vi "log analysis_gps.vi"() -> ()   [LabVIEW 2019] (continued)
-1.551528\t-0.373254\t-10.328419\t0.302000\t0.041000\n\t\n15:17:08.7\tlog_raw\tgps_raw\t#DUALANTENNAHEADINGA,USB3,0,50.0,FINESTEERING,2107,281846.700,02000000,d426,15824;SOL_COMPUTED,L1_FLOAT,-1.000000000,97.773071289,12.519289017,0.0,360.000000000,180.000000000,\"631T\",20,6,6,3,04,00,20,01*fc76e214\n\tsystem status\tnormal 2 27.800000 0 0\trobot status\t187.429657\t118.350310\t7.996000\t-1.404471\t-0.508241\t-9.481773\t0.290000\t0.043000\n\t\n15:17:09.2\tlog_raw\tgps_raw\t#DUALANTENNAHEADINGA,USB3,0,48.5,FINESTEERING,2107,281847.200,02000000,d426,15824;SOL_COMPUTED,L1_FLOAT,-1.000000000,99.566589355,2.463819742,0.0,360.000000000,180.000000000,\"631T\",20,6,6,3,04,00,20,01*aa8a8936\n\tsystem status\tnormal 2 27.900000 0 0\trobot status\t187.566793\t118.321024\t7.994500\t-1.416606\t-0.450416\t-8.715947\t0.329000\t-0.016000\n\t\n15:17:09.7\tlog_raw\tgps_raw\t#DUALANTENNAHEADINGA,USB3,0,48.5,FINESTEERING,2107,281847.700,02000000,d426,15824;SOL_COMPUTED,L1_FLOAT,-1.000000000,101.704925537,-0.791503906,0.0,360.000000000,180.000000000,\"631T\",21,6,6,3,04,00,20,01*ba1d7434\n\tsystem status\tnormal 2 28.000000 0 0\trobot status\t187.708819\t118.292371\t7.992200\t-1.444500\t-0.439049\t-8.038629\t0.312000\t-0.001000\n\t\n15:17:10.2\tlog_raw\tgps_raw\t#DUALANTENNAHEADINGA,USB3,0,48.0,FINESTEERING,2107,281848.200,02000000,d426,15824;SOL_COMPUTED,NARROW_FLOAT,-1.000000000,68.873619080,-13.291412354,0.0,268.060089111,180.000000000,\"631T\",21,7,7,5,04,00,20,03*0971a231\n\tsystem status\tnormal 2 28.000000 0 0\trobot status\t187.851802\t118.263763\t7.990800\t-1.419717\t-0.363643\t-7.607378\t0.249000\t0.089000\n\t\n15:17:10.7\tlog_raw\tgps_raw\t#DUALANTENNAHEADINGA,USB3,0,48.0,FINESTEERING,2107,281848.700,02000000,d426,15824;SOL_COMPUTED,NARROW_FLOAT,-1.000000000,68.326225281,-12.809478760,0.0,266.431640625,180.000000000,\"631T\",22,7,7,5,04,00,20,03*e2c6400d\n\tsystem status\tnormal 2 28.000000 0 0\trobot status\t187.993908\t118.234860\t7.989100\t-1.318472\t-0.217870\t-7.309537\t0.279000\t0.046000\n\t\n15:17:11.2\tlog_raw\tgps_raw\t#DUALANTENNAHEADINGA,USB3,0,49.0,FINESTEERING,2107,281849.200,02000000,d426,15824;SOL_COMPUTED,L1_FLOAT,-1.000000000,90.585990906,2.083147287,0.0,360.000000000,180.000000000,\"631T\",19,6,6,3,04,00,20,01*dc534f3f\n\tsystem status\tnormal 2 28.100000 0 0\trobot status\t188.136584\t118.206878\t7.987700\t-1.302740\t-0.167404\t-7.137371\t0.263000\t0.048000\n\t\n15:17:11.7\tlog_raw\tgps_raw\t\tsystem status\tnormal 2 28.100000 0 0\trobot status\t188.281681\t118.179408\t7.986200\t-1.424741\t-0.244800\t-7.144993\t0.355000\t-0.100000\n\t\n15:17:12.2\tlog_raw\tgps_raw\t\tsystem status\tnormal 2 28.100000 0 0\trobot status\t188.424376\t118.151727\t7.985000\t-1.444074\t-0.321672\t-7.277293\t0.280000\t0.006000\n\t\n15:17:12.7\tlog_raw\tgps_raw\t\tsystem status\tnormal 2 28.100000 0 0\trobot status\t188.565924\t118.124361\t7.984600\t-1.373448\t-0.224208\t-7.361017\t0.301000\t-0.011000\n\t\n15:17:13.2\tlog_raw\tgps_raw\t\tsystem status\tnormal 2 28.200000 0 0\trobot status\t188.708555\t118.095223\t7.983900\t-1.237162\t-0.173979\t-7.470326\t0.299000\t-0.027000\n\t\n15:17:13.7\tlog_raw\tgps_raw\t\tsystem status\tnormal 2 28.100000 0 0\trobot status\t188.846950\t118.066216\t7.984500\t-1.256970\t-0.201801\t-7.611888\t0.295000\t-0.025000\n\t\n15:17:14.2\tlog_raw\tgps_raw\t\tsystem status\tnormal 2 28.200000 0 0\trobot status\t188.990067\t118.035749\t7.985300\t-1.203931\t-0.250231\t-7.787271\t0.299000\t-0.026000\n\t\n15:17:14.7\tlog_raw\tgps_raw\t#DUALANTENNAHEADINGA,USB3,0,50.5,FINESTEERING,2107,281852.700,02000000,d426,15824;SOL_COMPUTED,L1_FLOAT,-1.000000000,102.741966248,-6.929687500,0.0,360.000000000,180.000000000,\"631T\",20,6,6,3,04,00,20,01*85f8aaaa\n\tsystem status\tnormal 2 28.100000 0 0\trobot status\t189.132338\t118.004982\t7.987500\t-1.054884\t-0.345405\t-7.976871\t0.298000\t-0.028000\n\t\n15:17:15.2\tlog_raw\tgps_raw\t#DUALANTENNAHEADINGA,USB3,0,48.0,FINESTEERING,2107,281853.200,02000000,d426,15824;SOL_COMPUTED,NARROW_FLOAT,-1.000000000,142.458068848,56.396076202,0.0,360.000000000,180.000000000,\"631T\",20,7,7,7,04,00,20,23*a5970788\n\tsystem status\tnormal 2 28.100000 0 0\trobot status\t189.287326\t117.973168\t7.989400\t-1.112733\t-0.467352\t-8.155902\t0.296000\t-0.018000\n\t\n15:17:15.7\tlog_raw\tgps_raw\t#DUALANTENNAHEADINGA,USB3,0,48.0,FINESTEERING,2107,281853.700,02000000,d426,15824;SOL_COMPUTED,NARROW_FLOAT,-1.000000000,133.951141357,46.090900421,0.0,360.000000000,180.000000000,\"631T\",20,7,7,7,04,00,20,23*158a3a24\n\tsystem status\tnormal 2 28.100000 0 0\trobot status\t189.431373\t117.943241\t7.991600\t-1.182526\t-0.406297\t-8.448718\t0.296000\t-0.020000\n\t\n15:17:16.2\tlog_raw\tgps_raw\t#INSPVAXA,USB3,0,49.5,FINESTEERING,2107,281854.250,02000000,471d,15824;INS_ALIGNMENT_COMPLETE,INS_RTKFIXED,37.37119259093,126.72297552525,7.9951,22.3000,-0.0458,0.2655,0.0156,-1.071259362,-0.181379499,98.712494459,0.4123,0.2982,0.5510,0.1098,0.0931,0.0772,0.1581,0.1591,4.8949,0f000001,0*3786ee92\n\tsystem status\tnormal 2 28.100000 0 0\trobot status\t189.594911\t117.907272\t7.995100\t-1.071259\t-0.181379\t-8.712494\t0.243000\t-0.107000\n\t\n15:17:16.7\tlog_raw\tgps_raw\t#INSPVAXA,USB3,0,49.5,FINESTEERING,2107,281854.750,02000000,471d,15824;INS_ALIGNMENT_COMPLETE,INS_RTKFIXED,37.37119229237,126.72297712322,7.9984,22.3000,-0.0524,0.2443,0.0048,-0.880696017,-0.044976851,99.111895186,0.4123,0.2982,0.5510,0.1098,0.0931,0.0772,0.1581,0.1591,4.8949,0f000001,0*8e46dd5f\n\tsystem status\tnormal 2 28.100000 0 0\trobot status\t189.736457\t117.874134\t7.998400\t-0.880696\t-0.044977\t-9.111895\t0.357000\t0.066000\n\t\n15:17:17.2\tlog_raw\tgps_raw\t#DUALANTENNAHEADINGA,USB3,0,49.0,FINESTEERING,2107,281855.200,02000000,d426,15824;SOL_COMPUTED,L1_FLOAT,-1.000000000,104.180160522,-12.584655762,0.0,360.000000000,180.000000000,\"631T\",18,6,6,3,04,00,20,01*befc2b24\n\tsystem status\tnormal 2 28.100000 0 0\trobot status\t189.862680\t117.843997\t8.000200\t-0.824988\t0.078029\t-9.657468\t0.282000\t-0.056000\n\t\n15:17:17.7\tlog_raw\tgps_raw\t#DUALANTENNAHEADINGA,USB3,0,49.0,FINESTEERING,2107,281855.700,02000000,d426,15824;SOL_COMPUTED,L1_FLOAT,-1.000000000,103.651336670,-10.938995361,0.0,360.000000000,180.000000000,\"631T\",18,6,6,3,04,00,20,01*040a1ee0\n\tsystem status\tnormal 2 28.000000 0 0\trobot status\t190.003868\t117.810762\t8.001400\t-1.003192\t0.238373\t-10.307968\t0.390000\t0.111000\n\t\n15:17:18.2\tlog_raw\tgps_raw\t#DUALANTENNAHEADINGA,USB3,0,50.0,FINESTEERING,2107,281856.200,02000000,d426,15824;SOL_COMPUTED,L1_FLOAT,-1.000000000,100.818984985,-10.711181641,0.0,360.000000000,180.000000000,\"631T\",17,6,6,3,04,00,20,01*31a96d86\n\tsystem status\tnormal 2 28.000000 0 0\trobot status\t190.147957\t117.774526\t8.001800\t-1.036464\t0.165737\t-11.023981\t0.342000\t0.033000\n\t\n15:17:18.7\tlog_raw\tgps_raw\t#DUALANTENNAHEADINGA,USB3,0,50.0,FINESTEERING,2107,281856.700,02000000,d426,15824;SOL_COMPUTED,L1_FLOAT,-1.000000000,103.587120056,-12.575134277,0.0,360.000000000,180.000000000,\"631T\",19,6,6,3,04,00,20,01*92b9a913\n\tsystem status\tnormal 2 28.000000 0 0\trobot status\t190.288239\t117.736616\t8.001900\t-0.987148\t0.177262\t-11.698662\t0.277000\t-0.056000\n\t\n15:17:19.2\tlog_raw\tgps_raw\t#DUALANTENNAHEADINGA,USB3,0,50.5,FINESTEERING,2107,281857.200,02000000,d426,15824;SOL_COMPUTED,NARROW_FLOAT,-1.000000000,171.941314697,65.361953735,0.0,360.000000000,180.000000000,\"631T\",19,5,5,5,04,00,20,03*703cece8\n\tsystem status\tnormal 2 28.000000 0 0\trobot status\t190.426855\t117.696346\t8.002000\t-0.898278\t0.171182\t-12.381846\t0.288000\t-0.043000\n\t\n15:17:19.7\tlog_raw\tgps_raw\t#DUALANTENNAHEADINGA,USB3,0,50.5,FINESTEERING,2107,281857.700,02000000,d426,15824;SOL_COMPUTED,NARROW_FLOAT,-1.000000000,164.009658813,63.451293945,0.0,360.000000000,180.000000000,\"631T\",20,5,5,5,04,00,20,03*1783c3a5\n\tsystem status\tnormal 2 28.000000 0 0\trobot status\t190.566426\t117.653463\t8.001500\t-0.881454\t0.086969\t-12.934182\t0.271000\t-0.059000\n\t\n15:17:20.2\tlog_raw\tgps_raw\t\tsystem status\tnormal 2 28.100000 0 0\trobot status\t190.706271\t117.610403\t8.001200\t-0.936167\t0.078921\t-13.431583\t0.286000\t-0.027000\n\t\n15:17:20.7\tlog_raw\tgps_raw\t\tsystem status\tnormal 2 28.100000 0 0\trobot status\t190.843432\t117.566420\t8.000900\t-0.762433\t0.230559\t-13.816991\t0.276000\t-0.043000\n\t\n15:17:21.2\tlog_raw\tgps_raw\t\tsystem status\tnormal 2 28.100000 0 0\trobot status\t190.981001\t117.522574\t8.001400\t-0.757985\t0.186515\t-14.116423\t0.318000\t0.024000\n\t\n15:17:21.7\tlog_raw\tgps_raw\t\tsystem status\tnormal 2 28.200000 0 0\trobot status\t191.119846\t117.477847\t8.003100\t-0.778462\t0.077157\t-14.338645\t0.273000\t-0.019000\n\t\n15:17:22.2\tlog_raw\tgps_raw\t\tsystem status\tnormal 2 28.100000 0 0\trobot status\t191.253862\t117.433724\t8.004800\t-0.857980\t0.194106\t-14.523909\t0.302000\t0.005000\n\t\n15:17:22.7\tlog_raw\tgps_raw\t\tsystem status\tnormal 2 28.100000 0 0\trobot status\t191.382625\t117.388434\t8.005800\t-0.734146\t0.154946\t-14.703088\t0.300000\t0.006000\n\t\n15:17:23.2\tlog_raw\tgps_raw\t\tsystem status\tnormal 2 28.100000 0 0\trobot status\t191.517770\t117.341159\t8.006800\t-0.593053\t0.103721\t-14.833385\t0.298000\t0.012000\n\t\n15:17:23.7\tlog_raw\tgps_raw\t\tsystem status\tnormal 2 28.100000 0 0\trobot status\t191.655942\t117.293810\t8.007700\t-0.579182\t0.136918\t-14.898404\t0.305000\t0.021000\n\t\n15:17:24.2\tlog_raw\tgps_raw\t\tsystem status\tnormal 2 28.100000 0 0\trobot status\t191.794529\t117.246111\t8.008900\t-0.513890\t0.130655\t-14.962199\t0.303000\t0.016000\n\t\n15:17:24.7\tlog_raw\tgps_raw\t\tsystem status\tnormal 2 28.100000 0 0\trobot status\t191.934007\t117.199632\t8.009600\t-0.626696\t0.037118\t-14.971745\t0.299000\t0.017000\n\t\n15:17:25.2\tlog_raw\tgps_raw\t\tsystem status\tnormal 2 28.100000 0 0\trobot status\t192.080157\t117.149836\t8.009200\t-0.638814\t-0.081979\t-14.950049\t0.368000\t-0.089000\n\t\n15:17:25.7\tlog_raw\tgps_raw\t\tsystem status\tnormal 2 28.100000 0 0\trobot status\t192.218407\t117.102393\t8.008000\t-0.698943\t-0.068914\t-14.782207\t0.293000\t0.043000\n\t\n15:17:26.2\tlog_raw\tgps_raw\t\tsystem status\tnormal 2 28.000000 0 0\trobot status\t192.353965\t117.056855\t8.007100\t-0.630226\t-0.049519\t-14.376017\t0.300000\t0.021000\n\t\n15:17:26.7\tlog_raw\tgps_raw\t\tsystem status\tnormal 2 28.000000 0 0\trobot status\t192.492478\t117.013307\t8.005800\t-0.518282\t0.005425\t-13.855730\t0.310000\t0.006000\n\t\n15:17:27.2\tlog_raw\tgps_raw\t#DUALANTENNAHEADINGA,USB3,0,46.0,FINESTEERING,2107,281865.200,02008000,d426,15824;SOL_COMPUTED,NARROW_FLOAT,-1.000000000,66.011009216,-7.448516846,0.0,202.896392822,180.000000000,\"631T\",18,7,7,5,04,00,20,03*493f8aff\n\tsystem status\tnormal 2 27.900000 0 0\trobot status\t192.633795\t116.970662\t8.002900\t-0.527369\t-0.067257\t-13.209593\t0.329000\t-0.021000\n\t\n15:17:27.7\tlog_raw\tgps_raw\t#DUALANTENNAHEADINGA,USB3,0,46.0,FINESTEERING,2107,281865.700,02008000,d426,15824;SOL_COMPUTED,NARROW_FLOAT,-1.000000000,65.260665894,-8.209533691,0.0,200.108810425,180.000000000,\"631T\",19,7,7,5,04,00,20,03*eb656687\n\tsystem status\tnormal 2 27.900000 0 0\trobot status\t192.772942\t116.929402\t8.000100\t-0.611867\t-0.146505\t-12.545248\t0.298000\t0.036000\n\t\n15:17:28.2\tlog_raw\tgps_raw\t#INSPVAXA,USB3,0,47.5,FINESTEERING,2107,281866.250,02008000,471d,15824;INS_ALIGNMENT_COMPLETE,INS_RTKFIXED,37.37118340706,126.72301312751,7.9981,22.3000,-0.0652,0.2808,0.0094,-0.679665296,-0.221411969,101.808618121,0.4126,0.2985,0.5507,0.1101,0.0933,0.0772,0.1577,0.1589,4.9112,0f000001,0*dd792aaa\n\tsystem status\tnormal 2 27.900000 0 0\trobot status\t192.925658\t116.887928\t7.998100\t-0.679665\t-0.221412\t-11.808618\t0.353000\t-0.059000\n\t\n15:17:28.7\tlog_raw\tgps_raw\t\tsystem status\tnormal 2 28.000000 0 0\trobot status\t193.051844\t116.857366\t7.996800\t-0.814985\t-0.169345\t-11.258005\t0.278000\t0.046000\n\t\n15:17:29.2\tlog_raw\tgps_raw\t#DUALANTENNAHEADINGA,USB3,0,49.0,FINESTEERING,2107,281867.200,02008000,d426,15824;SOL_COMPUTED,NARROW_FLOAT,-1.000000000,93.923080444,71.863670349,0.0,360.000000000,180.000000000,\"631T\",19,5,5,5,04,00,20,03*c6afd133\n\tsystem status\tnormal 2 28.000000 0 0\trobot status\t193.193872\t116.824950\t7.995200\t-0.948069\t-0.134343\t-10.713054\t0.411000\t-0.161000\n\t\n15:17:29.7\tlog_raw\tgps_raw\t#INSPVAXA,USB3,0,49.0,FINESTEERING,2107,281867.750,02008000,471d,15824;INS_ALIGNMENT_COMPLETE,INS_RTKFIXED,37.37118253054,126.72301786810,7.9941,22.3000,-0.0646,0.2786,0.0118,-0.915451137,-0.056618368,100.264591809,0.4127,0.2985,0.5509,0.1101,0.0933,0.0772,0.1576,0.1589,4.9117,0f000001,0*c2ba8d8d\n\tsystem status\tnormal 2 28.000000 0 0\trobot status\t193.345572\t116.790638\t7.994100\t-0.915451\t-0.056618\t-10.264592\t0.258000\t0.082000\n\t\n15:17:30.2\tlog_raw\tgps_raw\t#INSPVAXA,USB3,0,51.0,FINESTEERING,2107,281868.250,02000000,471d,15824;INS_ALIGNMENT_COMPLETE,INS_RTKFIXED,37.37118225307,126.72301943614,7.9928,22.3000,-0.0610,0.2887,0.0088,-0.787312923,0.119737638,100.099155235,0.4126,0.2984,0.5509,0.1099,0.0933,0.0772,0.1576,0.1589,4.9115,0f000001,0*f159e972\n\tsystem status\tnormal 2 28.100000 0 0\trobot status\t193.484466\t116.759840\t7.992800\t-0.787313\t0.119738\t-10.099155\t0.225000\t0.112000\n\t\n15:17:30.7\tlog_raw\tgps_raw\t\tsystem status\tnormal 2 28.100000 0 0\trobot status\t193.609834\t116.732428\t7.991600\t-0.785923\t0.297608\t-9.967972\t0.316000\t-0.042000\n\t\n15:17:31.2\tlog_raw\tgps_raw\t#INSPVAXA,USB3,0,50.5,FINESTEERING,2107,281869.250,02000000,471d,15824;INS_ALIGNMENT_COMPLETE,INS_RTKFIXED,37.37118172011,126.72302260767,7.9905,22.3000,-0.0480,0.2851,-0.0022,-0.913163720,0.118526501,100.070703566,0.4132,0.2986,0.5511,0.1100,0.0933,0.0772,0.1576,0.1589,4.9111,0f000001,0*65c3fc4b\n\tsystem status\tnormal 2 28.100000 0 0\trobot status\t193.765395\t116.700683\t7.990500\t-0.913164\t0.118527\t-10.070704\t0.248000\t0.069000\n\t\n15:17:31.7\tlog_raw\tgps_raw\t\tsystem status\tnormal 2 28.200000 0 0\trobot status\t193.890749\t116.675860\t7.989300\t-1.084192\t-0.039450\t-10.155472\t0.288000\t-0.004000\n\t\n15:17:32.2\tlog_raw\tgps_raw\t#INSPVAXA,USB3,0,52.5,FINESTEERING,2107,281870.250,02000000,471d,15824;INS_ALIGNMENT_COMPLETE,INS_RTKFIXED,37.37118119577,126.72302574832,7.9885,22.3000,-0.0604,0.2717,0.0033,-1.019669289,-0.207037760,100.231661614,0.4136,0.2987,0.5515,0.1101,0.0932,0.0772,0.1576,0.1589,4.9104,0f000001,0*d14905d5\n\tsystem status\tnormal 2 28.100000 0 0\trobot status\t194.043589\t116.642483\t7.988500\t-1.019669\t-0.207038\t-10.231662\t0.292000\t-0.016000\n\t\n15:17:32.7\tlog_raw\tgps_raw\t#INSPVAXA,USB3,0,52.5,FINESTEERING,2107,281870.750,02000000,471d,15824;INS_ALIGNMENT_COMPLETE,INS_RTKFIXED,37.37118091341,126.72302727970,7.9884,22.3000,-0.0515,0.2652,0.0073,-1.004852574,-0.259976693,100.327578359,0.4136,0.2987,0.5515,0.1101,0.0932,0.0772,0.1576,0.1589,4.9104,0f000001,0*d55530b8\n\tsystem status\tnormal 2 28.200000 0 0\trobot status\t194.179236\t116.611142\t7.988400\t-1.004853\t-0.259977\t-10.327578\t0.297000\t-0.023000\n\t\n15:17:33.2\tlog_raw\tgps_raw\t#INSPVAXA,USB3,0,45.5,FINESTEERING,2107,281871.250,02000000,471d,15824;INS_ALIGNMENT_COMPLETE,INS_RTKFIXED,37.37118063962,126.72302878446,7.9883,22.3000,-0.0590,0.2793,0.0105,-0.889527092,-0.301797073,100.467035019,0.4141,0.2986,0.5519,0.1101,0.0932,0.0772,0.1576,0.1590,4.9098,0f000001,0*e8d7f1cd\n\tsystem status\tnormal 2 28.100000 0 0\trobot status\t194.312525\t116.580753\t7.988300\t-0.889527\t-0.301797\t-10.467035\t0.303000\t-0.016000\n\t\n15:17:33.7\tlog_raw\tgps_raw\t#INSPVAXA,USB3,0,45.5,FINESTEERING,2107,281871.750,02000000,471d,15824;INS_ALIGNMENT_COMPLETE,INS_RTKFIXED,37.37118036572,126.72303032836,7.9872,22.3000,-0.0612,0.2876,0.0185,-0.836661662,-0.240967819,100.699833600,0.4141,0.2986,0.5519,0.1101,0.0932,0.0772,0.1576,0.1590,4.9098,0f000001,0*90542d7a\n\tsystem status\tnormal 2 28.100000 0 0\trobot status\t194.449281\t116.550351\t7.987200\t-0.836662\t-0.240968\t-10.699834\t0.296000\t-0.025000\n\t\n15:17:34.2\tlog_raw\tgps_raw\t#INSPVAXA,USB3,0,47.5,FINESTEERING,2107,281872.250,02000000,471d,15824;INS_ALIGNMENT_COMPLETE,INS_RTKFIXED,37.37118005951,126.72303202791,7.9860,22.3000,-0.0539,0.2801,0.0126,-0.854711157,-0.125084871,100.880826035,0.4137,0.2986,0.5517,0.1103,0.0932,0.0772,0.1576,0.1590,4.9098,0f000001,0*60ae78ad\n\tsystem status\tnormal 2 28.200000 0 0\trobot status\t194.599825\t116.516363\t7.986000\t-0.854711\t-0.125085\t-10.880826\t0.303000\t-0.017000\n\t\n15:17:34.7\tlog_raw\tgps_raw\t#INSPVAXA,USB3,0,47.5,FINESTEERING,2107,281872.750,02000000,471d,15824;INS_ALIGNMENT_COMPLETE,INS_RTKFIXED,37.37117976554,126.72303359862,7.9866,22.3000,-0.0553,0.2968,0.0085,-0.914496974,-0.073674951,101.177607301,0.4137,0.2986,0.5517,0.1103,0.0932,0.0772,0.1576,0.1590,4.9098,0f000001,0*11103b83\n\tsystem status\tnormal 2 28.100000 0 0\trobot status\t194.738955\t116.483733\t7.986600\t-0.914497\t-0.073675\t-11.177607\t0.312000\t-0.008000\n\t\n15:17:35.2\tlog_raw\tgps_raw\t#INSPVAXA,USB3,0,49.5,FINESTEERING,2107,281873.250,02000000,471d,15824;INS_ALIGNMENT_COMPLETE,INS_RTKFIXED,37.37117945174,126.72303522060,7.9882,22.3000,-0.0558,0.2814,0.0151,-0.882451939,-0.080219552,101.525271935,0.4183,0.2991,0.5543,0.1109,0.0933,0.0774,0.1576,0.1591,4.9099,0f000001,0*41fa168d\n\tsystem status\tnormal 2 28.100000 0 0\trobot status\t194.882628\t116.448903\t7.988200\t-0.882452\t-0.080220\t-11.525272\t0.328000\t0.023000\n\t\n15:17:35.7\tlog_raw\tgps_raw\t#INSPVAXA,USB3,0,49.5,FINESTEERING,2107,281873.750,02000000,471d,15824;INS_ALIGNMENT_COMPLETE,INS_RTKFIXED,37.37117913037,126.72303681813,7.9893,22.3000,-0.0511,0.2800,0.0116,-0.755728696,-0.179152544,102.026561049,0.4183,0.2991,0.5543,0.1109,0.0933,0.0774,0.1576,0.1591,4.9099,0f000001,0*23029c8c\n\tsystem status\tnormal 2 28.100000 0 0\trobot status\t195.024134\t116.413233\t7.989300\t-0.755729\t-0.179153\t-12.026561\t0.276000\t-0.062000\n\t\n15:17:36.2\tlog_raw\tgps_raw\t#INSPVAXA,USB3,0,50.5,FINESTEERING,2107,281874.250,02000000,471d,15824;INS_ALIGNMENT_COMPLETE,INS_RTKFIXED,37.37117879183,126.72303836597,7.9895,22.3000,-0.0480,0.2786,0.0068,-0.789121694,-0.227156967,102.683210616,0.4189,0.2989,0.5549,0.1108,0.0932,0.0774,0.1576,0.1590,4.9104,0f000001,0*be3d2619\n\tsystem status\tnormal 2 28.100000 0 0\trobot status\t195.161239\t116.375657\t7.989500\t-0.789122\t-0.227157\t-12.683211\t0.300000\t-0.036000\n\t\n15:17:36.7\tlog_raw\tgps_raw\t#INSPVAXA,USB3,0,50.5,FINESTEERING,2107,281874.750,02000000,471d,15824;INS_ALIGNMENT_COMPLETE,INS_RTKFIXED,37.37117842368,126.72303989869,7.9895,22.3000,-0.0579,0.2769,0.0167,-0.872070252,-0.189275732,103.407050365,0.4189,0.2989,0.5549,0.1108,0.0932,0.0774,0.1576,0.1590,4.9104,0f000001,0*e1385384\n\tsystem status\tnormal 2 28.000000 0 0\trobot status\t195.297005\t116.334794\t7.989500\t-0.872070\t-0.189276\t-13.407050\t0.316000\t-0.008000\n\t\n15:17:37.2\tlog_raw\tgps_raw\t#INSPVAXA,USB3,0,45.0,FINESTEERING,2107,281875.250,02000000,471d,15824;INS_ALIGNMENT_COMPLETE,INS_RTKFIXED,37.37117804326,126.72304144100,7.9897,22.3000,-0.0675,0.2838,0.0157,-0.838740489,-0.206654116,104.194830524,0.4175,0.2986,0.5544,0.1105,0.0931,0.0773,0.1576,0.1590,4.9111,0f000001,0*bfb33cdb\n\tsystem status\tnormal 2 28.000000 0 0\trobot status\t195.433621\t116.292571\t7.989700\t-0.838740\t-0.206654\t-14.194831\t0.346000\t0.038000\n\t\n15:17:37.7\tlog_raw\tgps_raw\t#INSPVAXA,USB3,0,45.0,FINESTEERING,2107,281875.750,02000000,471d,15824;INS_ALIGNMENT_COMPLETE,INS_RTKFIXED,37.37117766281,126.72304294804,7.9892,22.3000,-0.0643,0.2684,0.0190,-0.778611736,-0.142054720,104.951619331,0.4175,0.2986,0.5544,0.1105,0.0931,0.0773,0.1576,0.1590,4.9111,0f000001,0*c21e7554\n\tsystem status\tnormal 2 28.000000 0 0\trobot status\t195.567112\t116.250343\t7.989200\t-0.778612\t-0.142055\t-14.951619\t0.354000\t0.056000\n\t\n15:17:38.2\tlog_raw\tgps_raw\t#INSPVAXA,USB3,0,50.0,FINESTEERING,2107,281876.250,02000000,471d,15824;INS_ALIGNMENT_COMPLETE,INS_RTKFIXED,37.37117724261,126.72304445085,7.9872,22.3000,-0.0675,0.2686,0.0130,-0.693271652,-0.100470912,105.634006783,0.4157,0.2984,0.5536,0.1101,0.0930,0.0773,0.1576,0.1589,4.9121,0f000001,0*c817ed15\n\tsystem status\tnormal 2 28.000000 0 0\trobot status\t195.700228\t116.203704\t7.987200\t-0.693272\t-0.100471\t-15.634007\t0.254000\t-0.089000\n\t\n15:17:38.7\tlog_raw\tgps_raw\t#INSPVAXA,USB3,0,50.0,FINESTEERING,2107,281876.750,02000000,471d,15824;INS_ALIGNMENT_COMPLETE,INS_RTKFIXED,37.37117679224,126.72304598141,7.9858,22.3000,-0.0652,0.2661,0.0195,-0.773523356,-0.163286053,106.235029610,0.4157,0.2984,0.5536,0.1101,0.0930,0.0773,0.1576,0.1589,4.9121,0f000001,0*39dfe5ae\n\tsystem status\tnormal 2 28.100000 0 0\trobot status\t195.835803\t116.153717\t7.985800\t-0.773523\t-0.163286\t-16.235030\t0.265000\t-0.068000\n\t\n15:17:39.2\tlog_raw\tgps_raw\t#INSPVAXA,USB3,0,49.5,FINESTEERING,2107,281877.250,02000000,471d,15824;INS_ALIGNMENT_COMPLETE,INS_RTKFIXED,37.37117633133,126.72304748425,7.9850,22.3000,-0.0752,0.2541,0.0188,-0.756490501,-0.061250211,106.657417640,0.4141,0.2982,0.5527,0.1099,0.0930,0.0772,0.1576,0.1588,4.9134,0f000001,0*c347eea6\n\tsystem status\tnormal 2 28.100000 0 0\trobot status\t195.968922\t116.102560\t7.985000\t-0.756491\t-0.061250\t-16.657418\t0.277000\t-0.041000\n\t\n15:17:39.7\tlog_raw\tgps_raw\t#INSPVAXA,USB3,0,49.5,FINESTEERING,2107,281877.750,02000000,471d,15824;INS_ALIGNMENT_COMPLETE,INS_RTKFIXED,37.37117587185,126.72304894455,7.9858,22.3000,-0.0736,0.2566,0.0182,-0.691290554,0.115671295,106.950853651,0.4141,0.2982,0.5527,0.1099,0.0930,0.0772,0.1576,0.1588,4.9134,0f000001,0*bf0681f3\n\tsystem status\tnormal 2 28.100000 0 0\trobot status\t196.098273\t116.051562\t7.985800\t-0.691291\t0.115671\t-16.950854\t0.340000\t0.066000\n\t\n15:17:40.2\tlog_raw\tgps_raw\t#INSPVAXA,USB3,0,46.0,FINESTEERING,2107,281878.250,02000000,471d,15824;INS_ALIGNMENT_COMPLETE,INS_RTKFIXED,37.37117540642,126.72305040405,7.9858,22.3000,-0.0763,0.2617,0.0091,-0.690584467,0.289819266,107.189506996,0.4131,0.2981,0.5519,0.1099,0.0930,0.0771,0.1575,0.1588,4.9147,0f000001,0*24a15a5b\n\tsystem status\tnormal 2 28.100000 0 0\trobot status\t196.227553\t115.999903\t7.985800\t-0.690584\t0.289819\t-17.189507\t0.295000\t-0.001000\n\t\n15:17:40.7\tlog_raw\tgps_raw\t#INSPVAXA,USB3,0,46.0,FINESTEERING,2107,281878.750,02000000,471d,15824;INS_ALIGNMENT_COMPLETE,INS_RTKFIXED,37.37117493552,126.72305185756,7.9850,22.3000,-0.0783,0.2561,0.0099,-0.645148551,0.263210480,107.376836106,0.4131,0.2981,0.5519,0.1099,0.0930,0.0771,0.1575,0.1588,4.9147,0f000001,0*d1c1fe45\n\tsystem status\tnormal 2 28.100000 0 0\trobot status\t196.356302\t115.947638\t7.985000\t-0.645149\t0.263210\t-17.376836\t0.300000\t0.014000\n\t\n15:17:41.2\tlog_raw\tgps_raw\t#INSPVAXA,USB3,0,48.5,FINESTEERING,2107,281879.250,02000000,471d,15824;INS_ALIGNMENT_COMPLETE,INS_RTKFIXED,37.37117447448,126.72305323836,7.9839,22.3000,-0.0805,0.2449,0.0028,-0.594473310,0.228947195,107.558540148,0.4129,0.2981,0.5511,0.1100,0.0931,0.0771,0.1575,0.1588,4.9163,0f000001,0*ee394e1f\n\tsystem status\tnormal 2 28.100000 0 0\trobot status\t196.478611\t115.896466\t7.983900\t-0.594473\t0.228947\t-17.558540\t0.294000\t0.024000\n\t\n15:17:41.7\tlog_raw\tgps_raw\t#INSPVAXA,USB3,0,48.5,FINESTEERING,2107,281879.750,02000000,471d,15824;INS_ALIGNMENT_COMPLETE,INS_RTKFIXED,37.37117397984,126.72305472755,7.9828,22.3000,-0.0867,0.2510,0.0095,-0.498608617,0.229834885,107.620298376,0.4129,0.2981,0.5511,0.1100,0.0931,0.0771,0.1575,0.1588,4.9163,0f000001,0*d9024070\n\tsystem status\tnormal 2 28.100000 0 0\trobot status\t196.610521\t115.841566\t7.982800\t-0.498609\t0.229835\t-17.620298\t0.296000\t0.022000\n\t\n15:17:42.2\tlog_raw\tgps_raw\t#INSPVAXA,USB3,0,48.5,FINESTEERING,2107,281880.250,02000000,471d,15824;INS_ALIGNMENT_COMPLETE,INS_RTKFIXED,37.37117348165,126.72305623679,7.9838,22.3000,-0.0959,0.2852,0.0145,-0.523517116,0.173445039,107.625224225,0.4131,0.2981,0.5507,0.1100,0.0932,0.0771,0.1574,0.1588,4.9179,0f000001,0*6bf7a559\n\tsystem status\tnormal 2 28.100000 0 0\trobot status\t196.744207\t115.786271\t7.983800\t-0.523517\t0.173445\t-17.625224\t0.310000\t0.020000\n\t\n15:17:42.7\tlog_raw\tgps_raw\t#INSPVAXA,USB3,0,48.5,FINESTEERING,2107,281880.750,02000000,471d,15824;INS_ALIGNMENT_COMPLETE,INS_RTKFIXED,37.37117294431,126.72305789660,7.9831,22.3000,-0.0852,0.2698,0.0141,-0.555772515,0.079408991,107.669635072,0.4131,0.2981,0.5507,0.1100,0.0932,0.0771,0.1574,0.1588,4.9179,0f000001,0*1742ce26\n\tsystem status\tnormal 2 28.100000 0 0\trobot status\t196.891231\t115.726631\t7.983100\t-0.555773\t0.079409\t-17.669635\t0.270000\t0.074000\n\t\n15:17:43.2\tlog_raw\tgps_raw\t#INSPVAXA,USB3,0,47.5,FINESTEERING,2107,281881.250,02000000,471d,15824;INS_ALIGNMENT_COMPLETE,INS_RTKFIXED,37.37117244492,126.72305941240,7.9826,22.3000,-0.0757,0.2574,0.0112,-0.499737353,0.074053137,107.349848920,0.4135,0.2983,0.5505,0.1102,0.0933,0.0771,0.1574,0.1588,4.9194,0f000001,0*402f3f2b\n\tsystem status\tnormal 2 28.100000 0 0\trobot status\t197.025498\t115.671204\t7.982600\t-0.499737\t0.074053\t-17.349849\t0.308000\t0.012000\n\t\n15:17:43.7\tlog_raw\tgps_raw\t#INSPVAXA,USB3,0,47.5,FINESTEERING,2107,281881.750,02000000,471d,15824;INS_ALIGNMENT_COMPLETE,INS_RTKFIXED,37.37117196738,126.72306091172,7.9831,22.3000,-0.0783,0.2660,0.0186,-0.416436951,0.088853428,106.696307007,0.4135,0.2983,0.5505,0.1102,0.0933,0.0771,0.1574,0.1588,4.9194,0f000001,0*620f9249\n\tsystem status\tnormal 2 28.000000 0 0\trobot status\t197.158305\t115.618201\t7.983100\t-0.416437\t0.088853\t-16.696307\t0.280000\t0.053000\n\t\n15:17:44.2\tlog_raw\tgps_raw\t#INSPVAXA,USB3,0,44.5,FINESTEERING,2107,281882.250,02000000,471d,15824;INS_ALIGNMENT_COMPLETE,INS_RTKFIXED,37.37117150853,126.72306241559,7.9850,22.3000,-0.0608,0.2451,0.0066,-0.406550409,0.024677772,105.806071956,0.4138,0.2984,0.5505,0.1102,0.0933,0.0771,0.1573,0.1588,4.9208,0f000001,0*20d266fd\n\tsystem status\tnormal 2 27.900000 0 0\trobot status\t197.291515\t115.567272\t7.985000\t-0.406550\t0.024678\t-15.806072\t0.260000\t0.086000\n\t\n15:17:44.7\tlog_raw\tgps_raw\t\tsystem status\tnormal 2 27.800000 0 0\trobot status\t197.426255\t115.519167\t7.986500\t-0.414500\t0.008824\t-14.562240\t0.280000\t0.045000\n\t\n15:17:45.2\tlog_raw\tgps_raw\t#INSPVAXA,USB3,0,46.5,FINESTEERING,2107,281883.250,02000000,471d,15824;INS_ALIGNMENT_COMPLETE,INS_RTKFIXED,37.37117067641,126.72306545358,7.9876,22.3000,-0.0777,0.2473,0.0004,-0.446761173,0.141959315,103.301752998,0.4139,0.2985,0.5503,0.1102,0.0932,0.0771,0.1572,0.1587,4.9224,0f000001,0*34b690f3\n\tsystem status\tnormal 2 27.800000 0 0\trobot status\t197.560616\t115.474914\t7.987600\t-0.446761\t0.141959\t-13.301753\t0.296000\t0.047000\n\t\n15:17:45.7\tlog_raw\tgps_raw\t#INSPVAXA,USB3,0,46.5,FINESTEERING,2107,281883.750,02000000,471d,15824;INS_ALIGNMENT_COMPLETE,INS_RTKFIXED,37.37117030441,126.72306700472,7.9899,22.3000,-0.0617,0.2696,0.0265,-0.542142026,0.246764373,102.057621753,0.4139,0.2985,0.5503,0.1102,0.0932,0.0771,0.1572,0.1587,4.9224,0f000001,0*016cab57\n\tsystem status\tnormal 2 27.800000 0 0\trobot status\t197.698013\t115.433624\t7.989900\t-0.542142\t0.246764\t-12.057622\t0.300000\t0.040000\n\t\n15:17:46.2\tlog_raw\tgps_raw\t\tsystem status\tnormal 2 27.800000 0 0\trobot status\t197.838835\t115.393928\t7.992700\t-0.525404\t0.258786\t-10.934449\t0.303000\t0.031000\n\t\n15:17:46.7\tlog_raw\tgps_raw\t#INSPVAXA,USB3,0,48.0,FINESTEERING,2107,281884.750,02000000,471d,15824;INS_ALIGNMENT_COMPLETE,INS_RTKFIXED,37.37116962918,126.72307017450,7.9972,22.3000,-0.0537,0.2746,0.0133,-0.660873018,0.326948339,100.072587895,0.4139,0.2985,0.5502,0.1101,0.0931,0.0771,0.1571,0.1587,4.9240,0f000001,0*1475196f\n\tsystem status\tnormal 2 27.900000 0 0\trobot status\t197.978787\t115.358677\t7.997200\t-0.660873\t0.326948\t-10.072588\t0.297000\t0.022000\n\t\n15:17:47.2\tlog_raw\tgps_raw\t#INSPVAXA,USB3,0,46.5,FINESTEERING,2107,281885.250,02000000,471d,15824;INS_ALIGNMENT_COMPLETE,INS_RTKFIXED,37.37116932974,126.72307175980,8.0003,22.3000,-0.0553,0.2834,0.0118,-0.680106492,0.432078155,99.489485657,0.4137,0.2985,0.5500,0.1099,0.0931,0.0771,0.1571,0.1587,4.9256,0f000001,0*384d6b59\n\tsystem status\tnormal 2 27.900000 0 0\trobot status\t198.119210\t115.325441\t8.000300\t-0.680106\t0.432078\t-9.489486\t0.376000\t-0.105000\n\t\n15:17:47.7\tlog_raw\tgps_raw\t\tsystem status\tnormal 2 28.000000 0 0\trobot status\t198.262073\t115.293975\t8.002900\t-0.704926\t0.312956\t-9.072769\t0.353000\t-0.075000\n\t\n15:17:48.2\tlog_raw\tgps_raw\t#INSPVAXA,USB3,0,48.5,FINESTEERING,2107,281886.250,02000000,471d,15824;INS_ALIGNMENT_COMPLETE,INS_RTKFIXED,37.37116876559,126.72307497858,8.0043,22.3000,-0.0505,0.2700,0.0197,-0.630737523,0.236103622,98.774518000,0.4135,0.2984,0.5500,0.1099,0.0931,0.0771,0.1570,0.1587,4.9269,0f000001,0*06e1d073\n\tsystem status\tnormal 2 28.000000 0 0\trobot status\t198.404325\t115.262822\t8.004300\t-0.630738\t0.236104\t-8.774518\t0.360000\t-0.079000\n\t\n15:17:48.7\tlog_raw\tgps_raw\t#INSPVAXA,USB3,0,48.5,FINESTEERING,2107,281886.750,02000000,471d,15824;INS_ALIGNMENT_COMPLETE,INS_RTKFIXED,37.37116849518,126.72307655860,8.0058,22.3000,-0.0479,0.2894,0.0098,-0.729843639,0.253785173,98.685149837,0.4135,0.2984,0.5500,0.1099,0.0931,0.0771,0.1570,0.1587,4.9269,0f000001,0*6ed17162\n\tsystem status\tnormal 2 28.100000 0 0\trobot status\t198.544280\t115.232807\t8.005800\t-0.729844\t0.253785\t-8.685150\t0.290000\t0.003000\n\t\n15:17:49.2\tlog_raw\tgps_raw\t\tsystem status\tnormal 2 28.100000 0 0\trobot status\t198.686686\t115.201699\t8.008100\t-0.755823\t0.227491\t-8.731822\t0.351000\t-0.100000\n\t\n15:17:49.7\tlog_raw\tgps_raw\t#INSPVAXA,USB3,0,47.5,FINESTEERING,2107,281887.750,02000000,471d,15824;INS_ALIGNMENT_COMPLETE,INS_RTKFIXED,37.37116794085,126.72307975608,8.0103,22.3000,-0.0483,0.2817,0.0113,-0.853841864,0.188447476,98.810925200,0.4129,0.2983,0.5497,0.1100,0.0933,0.0771,0.1570,0.1587,4.9280,0f000001,0*b49a26d4\n\tsystem status\tnormal 2 28.100000 0 0\trobot status\t198.827508\t115.171278\t8.010300\t-0.853842\t0.188447\t-8.810925\t0.292000\t-0.009000\n\t\n15:17:50.2\tlog_raw\tgps_raw\t#INSPVAXA,USB3,0,50.0,FINESTEERING,2107,281888.250,02000000,471d,15824;INS_ALIGNMENT_COMPLETE,INS_RTKFIXED,37.37116766545,126.72308132013,8.0114,22.3000,-0.0457,0.2739,0.0034,-0.968854092,0.193025151,98.915996054,0.4125,0.2983,0.5497,0.1101,0.0935,0.0771,0.1571,0.1587,4.9288,0f000001,0*9b5c7e2f\n\tsystem status\tnormal 2 28.100000 0 0\trobot status\t198.966049\t115.140710\t8.011400\t-0.968854\t0.193025\t-8.915996\t0.297000\t-0.021000\n\t\n15:17:50.7\tlog_raw\tgps_raw\t\tsystem status\tnormal 2 28.100000 0 0\trobot status\t199.101129\t115.109772\t8.013100\t-0.954092\t0.130732\t-9.021357\t0.294000\t-0.023000\n\t\n15:17:51.2\tlog_raw\tgps_raw\t\tsystem status\tnormal 2 28.100000 0 0\trobot status\t199.241234\t115.075988\t8.015400\t-0.878188\t0.048960\t-9.203034\t0.298000\t-0.023000\n\t\n15:17:51.7\tlog_raw\tgps_raw\t#INSPVAXA,USB3,0,44.5,FINESTEERING,2107,281889.750,02000000,471d,15824;INS_ALIGNMENT_COMPLETE,INS_RTKFIXED,37.37116676559,126.72308604479,8.0182,22.3000,-0.0625,0.3054,0.0209,-0.972087805,-0.015873358,99.423505279,0.4122,0.2983,0.5496,0.1103,0.0935,0.0771,0.1571,0.1586,4.9293,0f000001,0*71ed46ba\n\tsystem status\tnormal 2 28.100000 0 0\trobot status\t199.384551\t115.040829\t8.018200\t-0.972088\t-0.015873\t-9.423505\t0.300000\t-0.031000\n\t\n15:17:52.2\tlog_raw\tgps_raw\t\tsystem status\tnormal 2 28.100000 0 0\trobot status\t199.535517\t115.004616\t8.020200\t-1.255751\t-0.122856\t-9.683240\t0.298000\t-0.025000\n\t\n15:17:52.7\tlog_raw\tgps_raw\t\tsystem status\tnormal 2 28.100000 0 0\trobot status\t199.684212\t114.966993\t8.021900\t-1.315549\t-0.233401\t-9.991614\t0.308000\t-0.016000\n\t\n15:17:53.2\tlog_raw\tgps_raw\t\tsystem status\tnormal 2 28.100000 0 0\trobot status\t199.830017\t114.928015\t8.023500\t-1.293198\t-0.204250\t-10.424533\t0.249000\t-0.095000\n\t\n15:17:53.7\tlog_raw\tgps_raw\t\tsystem status\tnormal 2 28.100000 0 0\trobot status\t199.973008\t114.887406\t8.025600\t-1.126159\t-0.339447\t-10.965064\t0.328000\t0.026000\n\t\n15:17:54.2\tlog_raw\tgps_raw\t#INSPVAXA,USB3,0,49.0,FINESTEERING,2107,281892.250,02000000,471d,15824;INS_ALIGNMENT_COMPLETE,INS_RTKFIXED,37.37116500965,126.72309429685,8.0266,22.3000,-0.0800,0.3032,0.0106,-1.000045816,-0.250485086,101.581647169,0.4117,0.2986,0.5496,0.1105,0.0935,0.0771,0.1571,0.1583,4.9290,0f000001,0*ebccc2b7\n\tsystem status\tnormal 2 28.000000 0 0\trobot status\t200.115505\t114.845930\t8.026600\t-1.000046\t-0.250485\t-11.581647\t0.256000\t-0.087000\n\t\n15:17:54.7\tlog_raw\tgps_raw\t#INSPVAXA,USB3,0,49.0,FINESTEERING,2107,281892.750,02000000,471d,15824;INS_ALIGNMENT_COMPLETE,INS_RTKFIXED,37.37116464489,126.72309588370,8.0261,22.3000,-0.0746,0.2919,0.0013,-0.966505403,-0.074133262,102.355415882,0.4117,0.2986,0.5496,0.1105,0.0935,0.0771,0.1571,0.1583,4.9290,0f000001,0*e99d934b\n\tsystem status\tnormal 2 28.000000 0 0\trobot status\t200.256066\t114.805444\t8.026100\t-0.966505\t-0.074133\t-12.355416\t0.291000\t-0.046000\n\t\n15:17:55.2\tlog_raw\tgps_raw\t\tsystem status\tnormal 2 28.000000 0 0\trobot status\t200.394623\t114.762679\t8.025200\t-0.883049\t0.047084\t-13.072897\t0.347000\t0.049000\n\t\n15:17:55.7\tlog_raw\tgps_raw\t#INSPVAXA,USB3,0,46.0,FINESTEERING,2107,281893.750,02000000,471d,15824;INS_ALIGNMENT_COMPLETE,INS_RTKFIXED,37.37116386545,126.72309901774,8.0239,22.3000,-0.0747,0.2810,0.0135,-0.903776454,0.116604665,103.770415844,0.4122,0.2987,0.5500,0.1103,0.0933,0.0771,0.1570,0.1582,4.9290,0f000001,0*419476b1\n\tsystem status\tnormal 2 28.000000 0 0\trobot status\t200.533674\t114.718931\t8.023900\t-0.903776\t0.116605\t-13.770416\t0.327000\t0.019000\n\t\n15:17:56.2\tlog_raw\tgps_raw\t\tsystem status\tnormal 2 28.100000 0 0\trobot status\t200.673888\t114.671391\t8.023100\t-0.780344\t-0.044040\t-14.304807\t0.486000\t0.267000\n\t\n15:17:56.7\tlog_raw\tgps_raw\t\tsystem status\tnormal 2 28.100000 0 0\trobot status\t200.812434\t114.622268\t8.023200\t-0.710034\t-0.024642\t-14.733065\t0.254000\t-0.089000\n\t\n15:17:57.2\tlog_raw\tgps_raw\t#INSPVAXA,USB3,0,46.0,FINESTEERING,2107,281895.250,02000000,471d,15824;INS_ALIGNMENT_COMPLETE,INS_RTKFIXED,37.37116255070,126.72310371548,8.0235,22.3000,-0.0988,0.2868,0.0058,-0.574989155,-0.045458111,105.108744593,0.4125,0.2988,0.5503,0.1099,0.0932,0.0771,0.1569,0.1580,4.9303,0f000001,0*d88c0d09\n\tsystem status\tnormal 2 28.100000 0 0\trobot status\t200.949792\t114.573004\t8.023500\t-0.574989\t-0.045458\t-15.108745\t0.228000\t-0.118000\n\t\n15:17:57.7\tlog_raw\tgps_raw\t\tsystem status\tnormal 2 28.100000 0 0\trobot status\t201.087357\t114.524139\t8.024100\t-0.529704\t-0.006010\t-15.372902\t0.306000\t0.004000\n\t\n15:17:58.2\tlog_raw\tgps_raw\t\tsystem status\tnormal 2 28.100000 0 0\trobot status\t201.217688\t114.475338\t8.024300\t-0.514330\t0.144194\t-15.609629\t0.296000\t-0.004000\n\t\n15:17:58.7\tlog_raw\tgps_raw\t\tsystem status\tnormal 2 28.200000 0 0\trobot status\t201.347593\t114.424740\t8.025000\t-0.475340\t0.273363\t-15.805007\t0.298000\t0.012000\n\t\n15:17:59.2\tlog_raw\tgps_raw\t\tsystem status\tnormal 2 28.200000 0 0\trobot status\t201.474451\t114.375806\t8.025600\t-0.465864\t0.335017\t-15.976555\t0.299000\t0.013000\n\t\n15:17:59.7\tlog_raw\tgps_raw\t\tsystem status\tnormal 2 28.200000 0 0\trobot status\t201.608394\t114.326106\t8.026200\t-0.486443\t0.340987\t-16.056357\t0.303000\t0.018000\n\t\n15:18:00.2\tlog_raw\tgps_raw\t\tsystem status\tnormal 2 28.100000 0 0\trobot status\t201.747627\t114.275240\t8.026100\t-0.403786\t0.192600\t-16.113922\t0.304000\t0.013000\n\t\n15:18:00.7\tlog_raw\tgps_raw\t\tsystem status\tnormal 2 28.100000 0 0\trobot status\t201.885548\t114.226129\t8.026300\t-0.337616\t0.019028\t-16.129286\t0.303000\t0.013000\n\t\n15:18:01.2\tlog_raw\tgps_raw\t\tsystem status\tnormal 2 28.100000 0 0\trobot status\t202.024097\t114.177325\t8.027000\t-0.406624\t-0.002105\t-16.116425\t0.363000\t-0.074000\n\t\n15:18:01.7\tlog_raw\tgps_raw\t\tsystem status\tnormal 2 28.100000 0 0\trobot status\t202.160021\t114.130047\t8.027700\t-0.461766\t-0.000322\t-15.795632\t0.309000\t0.022000\n\t\n15:18:02.2\tlog_raw\tgps_raw\t\tsystem status\tnormal 2 28.000000 0 0\trobot status\t202.294497\t114.084248\t8.028100\t-0.392250\t-0.007040\t-15.327034\t0.375000\t-0.080000\n\t\n15:18:02.7\tlog_raw\tgps_raw\t\tsystem status\tnormal 2 27.900000 0 0\trobot status\t202.423768\t114.043590\t8.028900\t-0.442481\t0.241505\t-14.716030\t0.299000\t0.029000\n\t\n15:18:03.2\tlog_raw\tgps_raw\t\tsystem status\tnormal 2 27.900000 0 0\trobot status\t202.558777\t114.003138\t8.030100\t-0.642243\t0.226998\t-13.917763\t0.243000\t0.112000\n\t\n15:18:03.7\tlog_raw\tgps_raw\t\tsystem status\tnormal 2 27.900000 0 0\trobot status\t202.692591\t113.963668\t8.031300\t-0.683100\t0.209136\t-13.072580\t0.242000\t0.114000\n\t\n15:18:04.2\tlog_raw\tgps_raw\t\tsystem status\tnormal 2 27.900000 0 0\trobot status\t202.825147\t113.926204\t8.032600\t-0.532598\t0.337286\t-12.368371\t0.289000\t0.034000\n\t\n15:18:04.7\tlog_raw\tgps_raw\t\tsystem status\tnormal 2 28.000000 0 0\trobot status\t202.958676\t113.891686\t8.033900\t-0.437583\t0.381203\t-11.744562\t0.317000\t-0.002000\n\t\n15:18:05.2\tlog_raw\tgps_raw\t\tsystem status\tnormal 2 28.000000 0 0\trobot status\t203.097769\t113.857773\t8.036000\t-0.533917\t0.240102\t-11.342279\t0.235000\t0.095000\n\t\n15:18:05.7\tlog_raw\tgps_raw\t\tsystem status\tnormal 2 28.000000 0 0\trobot status\t203.236225\t113.823358\t8.038800\t-0.629312\t0.189237\t-11.003329\t0.275000\t0.050000\n\t\n15:18:06.2\tlog_raw\tgps_raw\t\tsystem status\tnormal 2 28.100000 0 0\trobot status\t203.373447\t113.789446\t8.041100\t-0.652702\t0.062164\t-10.831688\t0.269000\t0.040000\n\t\n15:18:06.8\tlog_raw\tgps_raw\t\tsystem status\tnormal 2 28.100000 0 0\trobot status\t203.512144\t113.754262\t8.044000\t-0.497043\t0.065453\t-10.804375\t0.380000\t-0.132000\n\t\n15:18:07.3\tlog_raw\tgps_raw\t\tsystem status\tnormal 2 28.100000 0 0\trobot status\t203.649779\t113.719005\t8.046700\t-0.406621\t0.122364\t-10.878646\t0.287000\t0.005000\n\t\n15:18:07.8\tlog_raw\tgps_raw\t\tsystem status\tnormal 2 28.100000 0 0\trobot status\t203.785338\t113.684293\t8.049900\t-0.456072\t0.122610\t-10.993307\t0.301000\t-0.016000\n\t\n15:18:08.3\tlog_raw\tgps_raw\t\tsystem status\tnormal 2 28.100000 0 0\trobot status\t203.917369\t113.650686\t8.052400\t-0.671170\t0.192980\t-11.068263\t0.300000\t-0.021000\n\t\n15:18:08.8\tlog_raw\tgps_raw\t\tsystem status\tnormal 2 28.100000 0 0\trobot status\t204.052308\t113.614227\t8.054000\t-0.593540\t0.334523\t-11.176123\t0.302000\t-0.011000\n\t\n15:18:09.3\tlog_raw\tgps_raw\t\tsystem status\tnormal 2 28.100000 0 0\trobot status\t204.184653\t113.576596\t8.056100\t-0.505796\t0.403682\t-11.323692\t0.298000\t-0.022000\n\t\n15:18:09.8\tlog_raw\tgps_raw\t\tsystem status\tnormal 2 28.100000 0 0\trobot status\t204.324439\t113.537467\t8.059400\t-0.632981\t0.341223\t-11.543184\t0.297000\t-0.023000\n\t\n15:18:10.3\tlog_raw\tgps_raw\t\tsystem status\tnormal 2 28.100000 0 0\trobot status\t204.468485\t113.496061\t8.062500\t-0.791445\t0.271242\t-11.755783\t0.297000\t-0.020000\n\t\n15:18:10.8\tlog_raw\tgps_raw\t\tsystem status\tnormal 2 28.100000 0 0\trobot status\t204.606800\t113.454791\t8.066300\t-0.973900\t0.283318\t-12.051295\t0.302000\t-0.014000\n\t\n15:18:11.3\tlog_raw\tgps_raw\t\tsystem status\tnormal 2 28.100000 0 0\trobot status\t204.746824\t113.411054\t8.070600\t-0.829760\t0.324767\t-12.387887\t0.313000\t-0.004000\n\t\n15:18:11.8\tlog_raw\tgps_raw\t\tsystem status\tnormal 2 28.100000 0 0\trobot status\t204.887401\t113.367932\t8.073700\t-0.772847\t0.310907\t-12.805151\t0.234000\t-0.122000\n\t\n15:18:12.3\tlog_raw\tgps_raw\t\tsystem status\tnormal 2 28.100000 0 0\trobot status\t205.024753\t113.324627\t8.077000\t-0.858536\t0.429761\t-13.257938\t0.277000\t-0.056000\n\t\n15:18:12.8\tlog_raw\tgps_raw\t\tsystem status\tnormal 2 28.100000 0 0\trobot status\t205.160638\t113.279510\t8.081400\t-0.891338\t0.356606\t-13.745466\t0.283000\t-0.039000\n\t\n15:18:13.3\tlog_raw\tgps_raw\t\tsystem status\tnormal 2 28.100000 0 0\trobot status\t205.297090\t
